vi "test vi conpane specs.vi"() -> ()   [LabVIEW 2009]
panel:
  out "VI fits specs?":bool
  in  "vi path":path
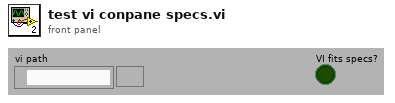
[diagram p1: front panel]
types:
  T1 = cluster{"Datatype":variant, "Control (T)":bool}[]
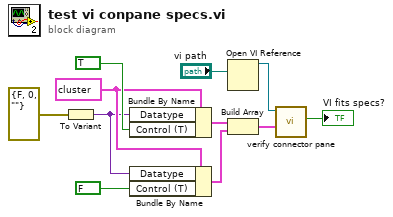
[diagram p0: block diagram]
diagram:
  w7 = cluster{"Datatype":variant, "Control (T)":bool} {"Datatype"=variant, "Control (T)"=TRUE} ("Terminal")
  n1 = To Variant(anything=errorcluster {"status"=FALSE, "code"=0, "source"=""} ("error in (no error)")) -> (Variant=w6:variant)
  n2 = Bundle By Name(cluster=w7, "Datatype"=w6, "Control (T)"=TRUE) -> (w3:cluster{"Datatype":variant, "Control (T)":bool})
  n3 = Bundle By Name(cluster=w7, "Datatype"=w6, "Control (T)"=FALSE) -> (w4:cluster{"Datatype":variant, "Control (T)":bool})
  n4 = Open VI Reference(vi path="vi path") -> (vi reference=w10:refnum<vi>)  [unwired: 5 in, 1 out]
  n5 = Build Array(w3, w4) -> (w2:T1)
  n6 = call "verify connector pane.vi"("Control pane terminals"=w2, "VI"=w10) -> ("VI fits specs?"=→"VI fits specs?":bool)  [unwired: 9 in]
